vi "ZoomInOut.vi"(0 "Map in":refnum<vi>, 1 "Direction":enum16{"Out", "In"}(ring), 2 "Zoom diff":dbl, 3 "Image Size":cluster{dbl, dbl}, 4 "Iterations":i32) -> (5 "Map out":refnum<vi>)   [LabVIEW 2014]
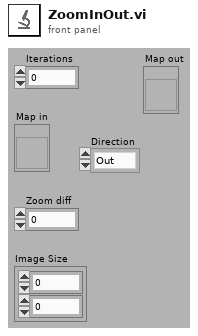
[diagram p1: front panel]
types:
  T1 = typedef "LVPointTypeDef.ctl" = cluster{"Horizontal":i16, "Vertical":i16}
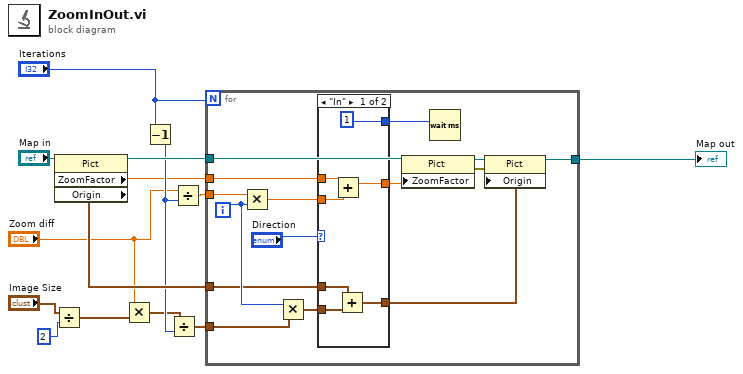
[diagram p0: block diagram]
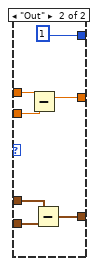
[diagram p2: hidden frame]
diagram:
  n1 = Divide(x="Image Size", y=2) -> (x/y=w3:cluster{dbl, dbl})
  n2 = property class="Pict"(reference="Map in") -> (reference out=w9:refnum<vi>, "ZoomFactor"=w4:sgl, "Origin"=w12:T1)  [unwired: 1 in, 1 out]
  n3 = Multiply(x="Zoom diff", y=w3) -> (x*y=w2:cluster{dbl, dbl})
  n4 = Decrement(x="Iterations") -> (x-1=w6:i32)
  n5 = Divide(x=w2, y=w6) -> (x/y=w5:cluster{dbl, dbl})
  n6 = Divide(x="Zoom diff", y=w6) -> (x/y=w11:dbl)
  n7 = for {
    N: "Iterations" -> [_]
    tunnel: w11 -> [w29]
    tunnel: w9 -> [w28]
    tunnel: w4 -> [w27]
    tunnel: [w19] -> w13
    tunnel: w5 -> [w22]
    tunnel: w12 -> [w21]
    i -> [w23]
    n8 = Multiply(x=w29, y=w23) -> (x*y=w26:dbl)
    n9 = Multiply(x=w23, y=w22) -> (x*y=w20:cluster{dbl, dbl})
    n10 = case shown="\"In\"" "Direction" {
      tunnel: w27 -> [w36 w43]
      tunnel: w26 -> [w35 w42]
      tunnel: [w34 w41] -> w24
      tunnel: w21 -> [w33 w40]
      tunnel: w20 -> [w32 w39]
      tunnel: [w31 w38] -> w18
      tunnel: [u32 1 ("milliseconds to wait") u32 1 ("milliseconds to wait")] -> w15
      frame "In" {
        n11 = Add(x=w36, y=w35) -> (x+y=w34:dbl)
        n12 = Add(x=w33, y=w32) -> (x+y=w31:cluster{dbl, dbl})
      }
      frame "Out" {
        n13 = Subtract(x=w43, y=w42) -> (x-y=w41:dbl)
        n14 = Subtract(x=w40, y=w39) -> (x-y=w38:cluster{dbl, dbl})
      }
    }
    n15 = property class="Pict"(reference=w28, "ZoomFactor"=w24) -> (reference out=w25:refnum<vi>, error out=w17:errorcluster)  [unwired: 1 in]
    n16 = Wait (ms)(milliseconds to wait=w15) -> ()  [unwired: 1 out]
    n17 = property class="Pict"(reference=w25, error in=w17, "Origin"=w18) -> (reference out=w19:refnum<vi>)  [unwired: 1 out]
  }
  "Map out" <- w13
